vi "cw_1_9.vi"() -> ()   [LabVIEW 2022 SP3]
panel:
  in  "Set Limits":cluster{dbl, dbl}(slide) scale=0.0..1000.0
  out "Number in Range":bool
  in  "Temp":dbl(slide) scale=0.0..1000.0
  out "Lower Limit":dbl(knob) scale=0.0..1000.0
  out "Upper Limit":dbl(knob) scale=0.0..1000.0
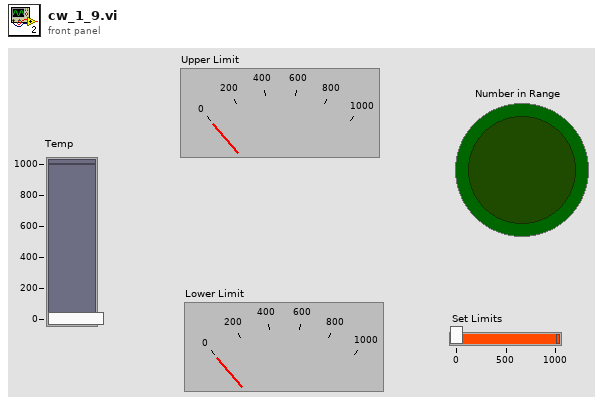
[diagram p1: front panel]
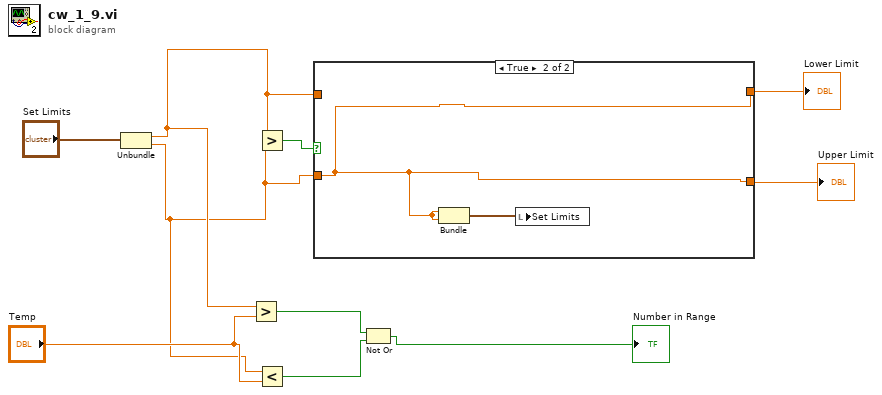
[diagram p0: block diagram]
diagram:
  n1 = Unbundle("Set Limits") -> (w5:dbl, w4:dbl)
  n2 = Greater?(x=w5, y="Temp") -> (0:w3:bool)
  n3 = Greater?(x=w5, y=w4) -> (0:w9:bool)
  n4 = Less?(x=w4, y="Temp") -> (x < y?=w2:bool)
  n5 = case shown="True" w9 {
    tunnel: w4 -> [w12 w13]
    tunnel: [w12 w13] -> w8
    tunnel: w5 -> [w11 _]
    tunnel: [w11 w13] -> w7
    frame False {
    }
    frame True {
      n6 = Bundle(w13, w13) -> (w14:cluster{dbl, dbl})  [unwired: 1 in]
      n7 = local write "Set Limits"(w14) -> ()
    }
  }
  "Upper Limit" <- w8
  "Lower Limit" <- w7
  n8 = Not Or(1:w2, 2:w3) -> (0:→"Number in Range":bool)
